vi "Dec_Num_to_Character.vi"(11 "Decimal Number":i32=10) -> (3 "Output String":string="A")   [LabVIEW 2011]
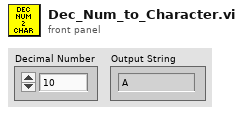
[diagram p1: front panel]
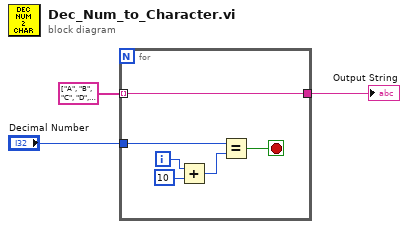
[diagram p0: block diagram]
diagram:
  n1 = for {
    tunnel: string[] ["A", "B", "C", "D", "E", "F", "G", "H", "I", "J", "K", "L", "M", "N", "O", "P", "Q", "R", "S", "T", "U", "V", "W", "X", "Y", "Z"] -> [w4] mode=indexing
    tunnel: "Decimal Number" -> [w9]
    tunnel: [w4] -> w1
    i -> [w8]
    stop <- w5 stop-if-true
    n2 = Add(x=w8, y=10) -> (x+y=w6:i32)
    n3 = Equal?(x=w9, y=w6) -> (x = y?=w5:bool)
  }
  "Output String" <- w1
